vi "VALEW_ATC_Calc Bath Temp.vi"(0 "V(bath cold)":dbl, 5 "V(bath)":dbl, 7 "T(cold inlet)":dbl, 9 "V(bath hot)":dbl, 11 "T(hot inlet)":dbl) -> (8 "T(bath)":dbl)   [LabVIEW 2016, in "TLMB.lvlib"]
uses:
  Projects/TLMB.lvlib
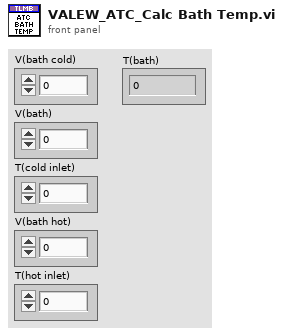
[diagram p1: front panel]
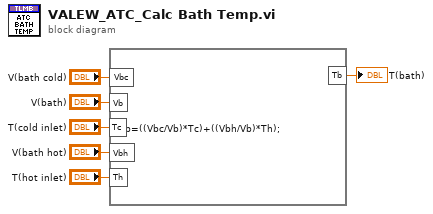
[diagram p0: block diagram]
diagram:
  n1 = formula code="Tb=((Vbc/Vb)*Tc)+((Vbh/Vb)*Th);"("Vbc"="V(bath cold)", "Vb"="V(bath)", "Tc"="T(cold inlet)", "Vbh"="V(bath hot)", "Th"="T(hot inlet)") -> ("Tb"=→"T(bath)":dbl)
